vi "DataProcessingDraft.vi"() -> ()   [LabVIEW 2011]
uses:
  olin-sail-bot/Software/2-Think/2 Typedefs/logger data.ctl
  olin-sail-bot/Software/2-Think/2 Typedefs/Which Boat.ctl
  olin-sail-bot/Software/2-Think/2 Typedefs/UTM Location.ctl
  olin-sail-bot/Software/2-Think/2 Typedefs/heading.ctl
  olin-sail-bot/Software/2-Think/2 Typedefs/rate of turn.ctl
  olin-sail-bot/Software/2-Think/2 Typedefs/robot velocity.ctl
  olin-sail-bot/Software/2-Think/2 Typedefs/pitch and roll.ctl
  olin-sail-bot/Software/2-Think/2 Typedefs/generalized sensor status.ctl
  olin-sail-bot/Software/2-Think/2 Typedefs/indicator LED.ctl
  olin-sail-bot/Software/2-Think/2 Typedefs/apparent wind direction.ctl
  olin-sail-bot/Software/2-Think/2 Typedefs/apparent wind speed.ctl
  olin-sail-bot/Software/2-Think/2 Typedefs/absolute wind direction.ctl
  olin-sail-bot/Software/2-Think/2 Typedefs/absolute wind speed.ctl
  olin-sail-bot/Software/0x2-OCU-Think Comm/0x2 Typedefs/Current Waypoint.ctl
  olin-sail-bot/Software/2-Think/2 Typedefs/UTM Circle.ctl
  olin-sail-bot/Software/2-Think/2 Typedefs/rudder angle.ctl
  olin-sail-bot/Software/2-Think/2 Typedefs/sail setpt.ctl
  olin-sail-bot/Software/0x2-OCU-Think Comm/0x2 Typedefs/manual override.ctl
  olin-sail-bot/Software/2-Think/2 Typedefs/setpoints to boat.ctl
panel:
  in  "Stop Viewing Data":bool
  in  "Choose graph to display":T1(tab)
  in  "Max Frequency":dbl
  out "Code Speed":cluster{i32[], dbl[]}[](graph)
  out "Battery Voltage":cluster{i32[], dbl[]}(graph)
  in  "Max Velocity":dbl
  out "Velocity":cluster{i32[], dbl[]}[](graph)
  in  "Max Angle":dbl
  out "Headings":cluster{i32[], dbl[]}[](graph)
  out "Rudder":cluster{i32[], dbl[]}(graph)
  out "Sail":cluster{i32[], dbl[]}(graph)
  in  "Data Log":T2 {"Current Waypoint Coords"."North" format="%#_10f"; "Current Waypoint Coords"."East" format="%#_8f"; "Robot Pitch/Roll"."Roll" format="%05.1f"; "Robot Pitch/Roll"."Pitch" format="%05.1f"; "Robot\nRate of Turn" format="%05.1f"; "Robot\nHeading" format="%05.1f"; "Robot UTM Location"."North" format="%#_10f"; "Robot UTM Location"."East" format="%#_8f"}
  # "Act and network frequency are always 0.\nAs far as I can tell, network frequency is never set, so of course it's 0.\nAct, while set, is in a sequence structure where the first frame has a while loop that only ends if we e-stop, so it'll never get set."
  # "Where Am I?"
  # "Path Planning"
  # "From Planning Functions"
  # "(this is not a cluster because subitems\nare generated in parallel code)"
  # "How Am I?"
  # "What's Around Me?"
  # "As Measured"
  # "As Measured"
  # "Loop Rates"
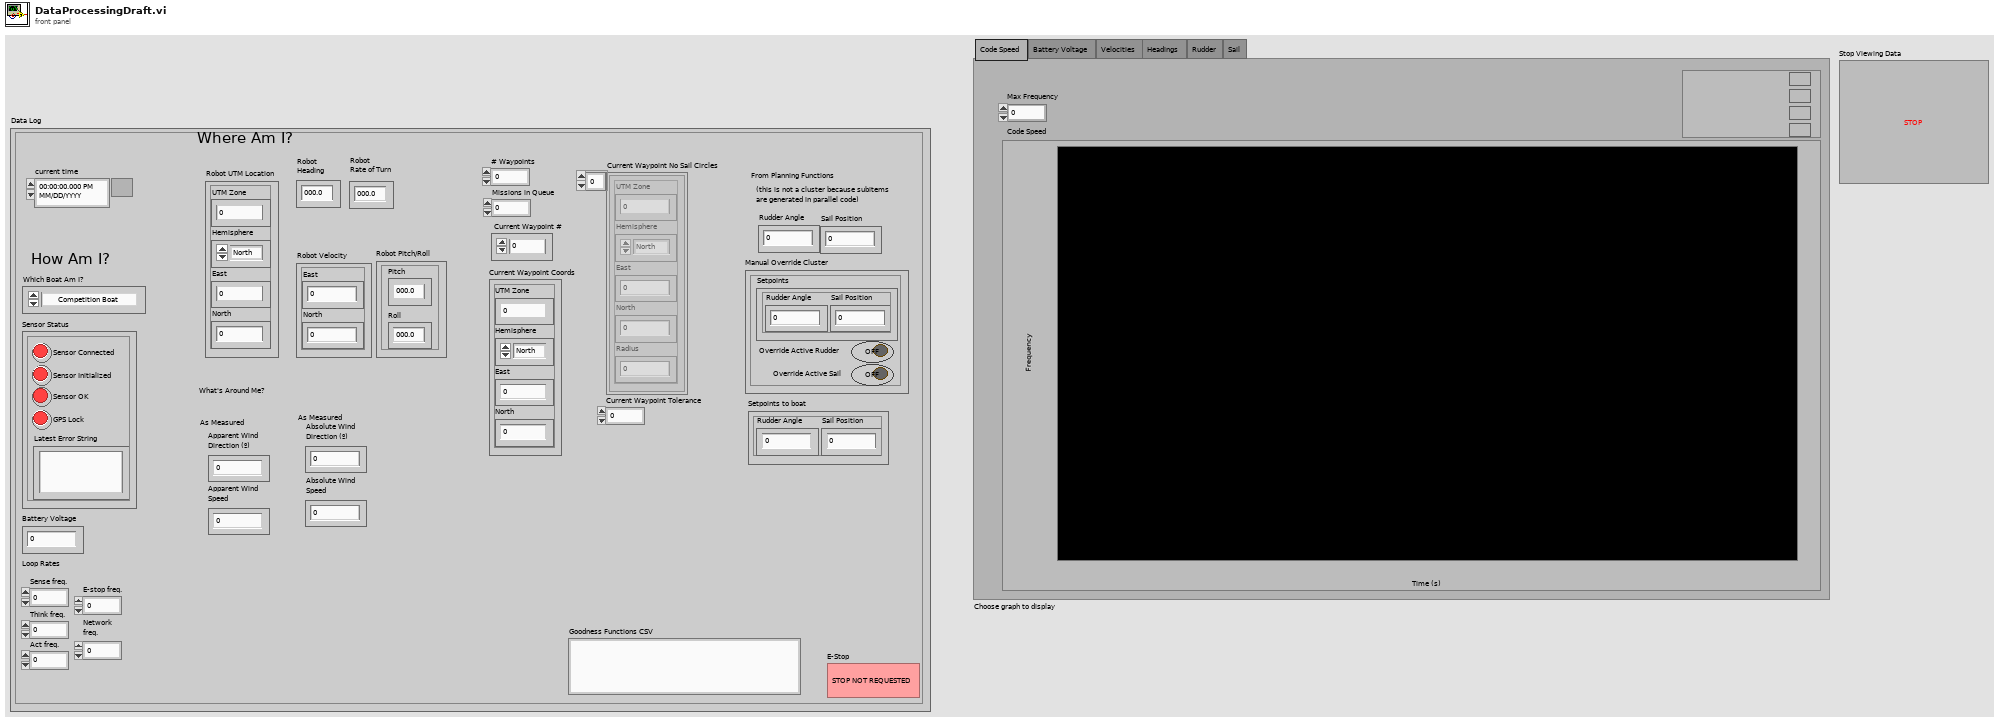
[diagram p1: front panel]
types:
  T1 = enum32{"Code Speed", "Battery Voltage", "Velocities", "Headings", "Rudder", "Sail"}
  T2 = typedef "logger data.ctl" = cluster{"current time":timestamp, "Which Boat Am I?":T3, "Robot UTM Location":T4, "Robot\nHeading ":T5, "Robot\nRate of Turn":T6, "Robot Velocity":T7, "Robot Pitch/Roll":T8, "Sensor Status":T9, "Battery Voltage":dbl, "Sense freq.":dbl, "Think freq.":dbl, "Act freq.":dbl, "E-stop freq.":dbl, "Network \nfreq.":dbl, "Apparent Wind\nDirection (º)":T11, "Apparent Wind\nSpeed":T12, "Absolute Wind\nDirection (º)":T13, "Absolute Wind\nSpeed":T14, "Missions in Queue":i32, "# Waypoints":i32, " Current Waypoint #":T15, "Current Waypoint Coords":T4, "Current Waypoint Tolerance":dbl, "Current Waypoint No Sail Circles":T16[], "Rudder Angle":T17, "Sail Position":T18, "Manual Override Cluster":T19, "Setpoints to boat":T20, "E-Stop":bool, "Goodness Functions CSV":string}
  T3 = typedef "Which Boat.ctl" = enum16{"Competition Boat", "Small RC", "Simulation"}
  T4 = typedef "UTM Location.ctl" = cluster{"UTM Zone":dbl, "Hemisphere":enum16{"North", "South"}, "East":dbl, "North":dbl}
  T5 = typedef "heading.ctl" = dbl
  T6 = typedef "rate of turn.ctl" = dbl
  T7 = typedef "robot velocity.ctl" = cluster{"East":dbl, "North":dbl}
  T8 = typedef "pitch and roll.ctl" = cluster{"Pitch":dbl, "Roll":dbl}
  T9 = typedef "generalized sensor status.ctl" = cluster{"Sensor Connected":T10, "Sensor Initialized":T10, "Sensor OK":T10, "Latest Error String":string, "GPS Lock":T10}
  T10 = typedef "indicator LED.ctl" = bool
  T11 = typedef "apparent wind direction.ctl" = dbl
  T12 = typedef "apparent wind speed.ctl" = dbl
  T13 = typedef "absolute wind direction.ctl" = dbl
  T14 = typedef "absolute wind speed.ctl" = dbl
  T15 = typedef "Current Waypoint.ctl" = i32
  T16 = typedef "UTM Circle.ctl" = cluster{"UTM Zone":dbl, "Hemisphere":enum16{"North", "South"}, "East":dbl, "North":dbl, "Radius":dbl}
  T17 = typedef "rudder angle.ctl" = dbl
  T18 = typedef "sail setpt.ctl" = dbl
  T19 = typedef "manual override.ctl" = cluster{"Override Active Rudder":bool, "Setpoints":T20, "Override Active Sail":bool}
  T20 = typedef "setpoints to boat.ctl" = cluster{"Sail Position":T18, "Rudder Angle":T17}
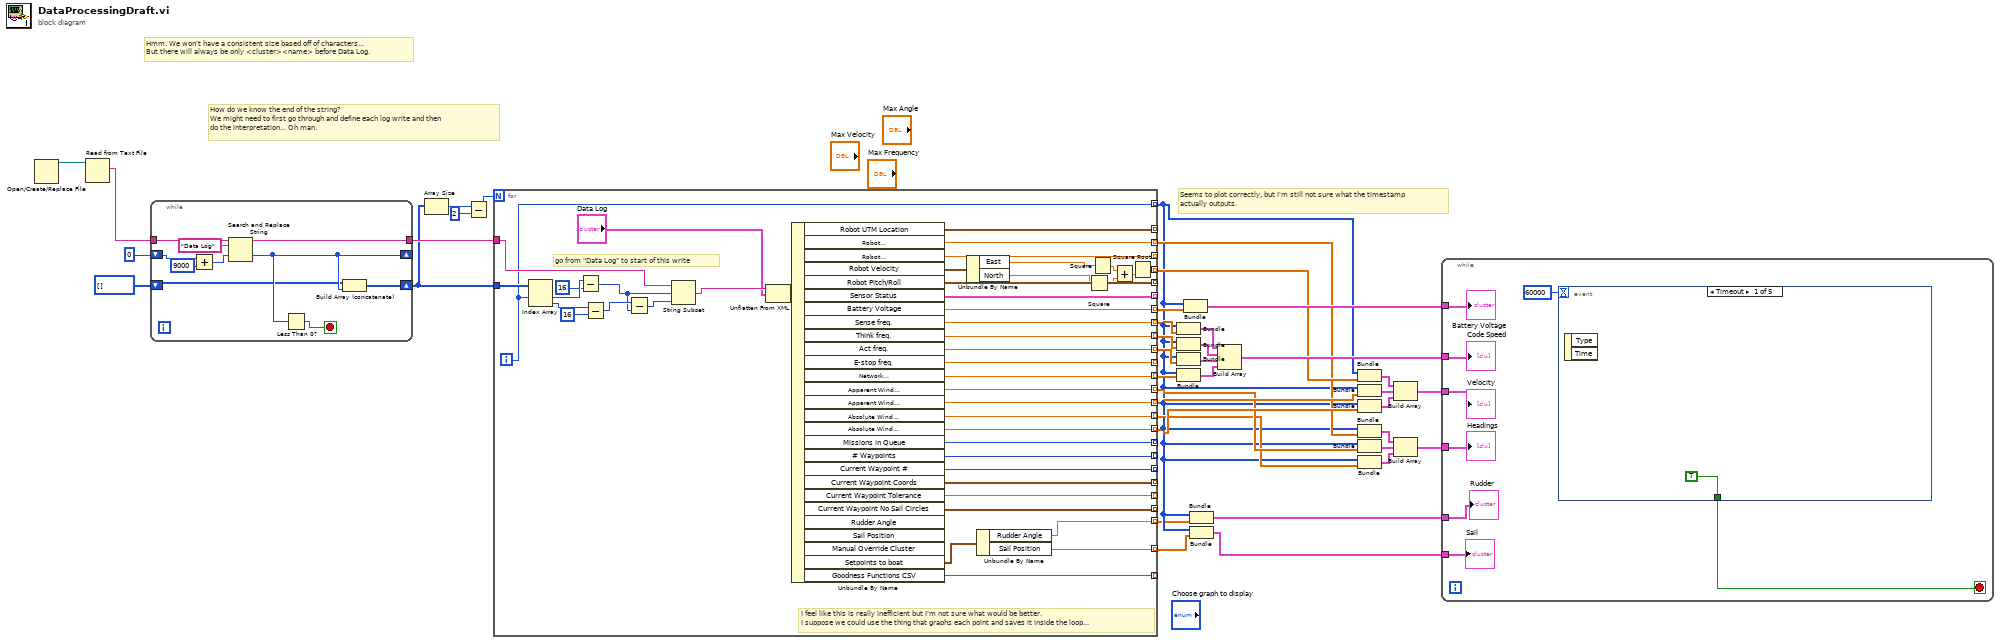
[diagram p0: block diagram]
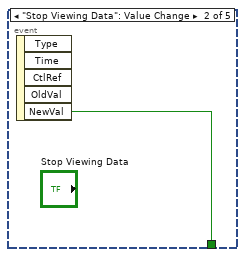
[diagram p2: hidden frame]
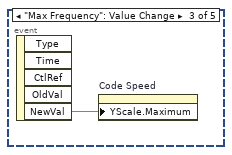
[diagram p3: hidden frame]
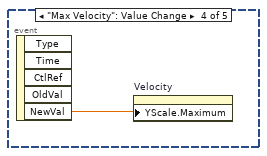
[diagram p4: hidden frame]
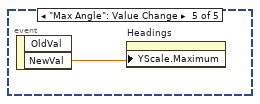
[diagram p5: hidden frame]
diagram:
  # "Seems to plot correctly, but I'm still not sure what the timestamp\nactually outputs."
  # "How do we know the end of the string?\nWe might need to first go through and define each log write and then\ndo the interpretation... Oh man."
  # "Hmm. We won't have a consistent size based off of characters...\nBut there will always be only <cluster><name> before Data Log."
  n1 = Open/Create/Replace File() -> (refnum out=w39:refnum<file>)  [unwired: 6 in, 2 out]
  n2 = Read from Text File(file (use dialog)=w39) -> (text=w38:string)  [unwired: 3 in, 3 out]
  n3 = while {
    tunnel: w38 -> [w48]
    shift-right: [w43] -> _
    shift-left: 0 ("offset past replacement") -> [w47]
    shift-right: [w42] -> w34
    shift-left: i32[] [] -> [w41]
    tunnel: [w40] -> w35
    stop <- w44 stop-if-true
    n4 = Add(x=w47, y=9000) -> (x+y=w45:i32)
    n5 = Search and Replace String(input string=w48, search string="Data Log", offset=w45) -> (result string=w40:string, offset past replacement=w43:i32)  [unwired: 5 in, 2 out]
    n6 = Less Than 0?(x=w43) -> (x < 0?=w44:bool)
    n7 = Build Array (concatenate)(w41, w43) -> (w42:i32[])
  }
  n8 = Array Size(array=w34) -> (size(s)=w33:i32)
  n9 = Subtract(x=w33, y=2) -> (x-y=w32:i32)
  n10 = for {
    N: w32 -> [_]
    tunnel: w34 -> [w86]
    tunnel: w35 -> [w89]
    tunnel: [w82] -> _ mode=indexing
    tunnel: [w81] -> w9 mode=indexing
    tunnel: [w80] -> _ mode=indexing
    tunnel: [w79] -> _ mode=indexing
    tunnel: [w78] -> _ mode=indexing
    tunnel: [w77] -> w20 mode=indexing
    tunnel: [w76] -> w18 mode=indexing
    tunnel: [w75] -> w17 mode=indexing
    tunnel: [w74] -> w16 mode=indexing
    tunnel: [w73] -> _ mode=indexing
    tunnel: [w72] -> w15 mode=indexing
    tunnel: [w71] -> w8 mode=indexing
    tunnel: [w70] -> w12 mode=indexing
    tunnel: [w69] -> w7 mode=indexing
    tunnel: [w68] -> w11 mode=indexing
    tunnel: [w67] -> _ mode=indexing
    tunnel: [w66] -> _ mode=indexing
    tunnel: [w65] -> _ mode=indexing
    tunnel: [w64] -> _ mode=indexing
    tunnel: [w63] -> _ mode=indexing
    tunnel: [w62] -> _ mode=indexing
    tunnel: [w61] -> _ mode=indexing
    tunnel: [w60] -> w6 mode=indexing
    tunnel: [w53] -> w13 mode=indexing
    tunnel: [w51] -> w4 mode=indexing
    tunnel: [w50] -> w3 mode=indexing
    i -> [w60]
    # "I feel like this is really inefficient but I'm not sure what would be better.\nI suppose we could use the thing that graphs each point and saves it inside the loop..."
    # "go from \"Data Log\" to start of this write"
    n11 = Index Array(array=w86, index #1=w60) -> (element #1=w94:i32, element #2=w92:i32)  [unwired: 1 in]
    n12 = Subtract(x=w94, y=16) -> (x-y=w87:i32)
    n13 = Subtract(x=w92, y=16) -> (x-y=w90:i32)
    n14 = Subtract(x=w90, y=w87) -> (x-y=w88:i32)
    n15 = String Subset(string=w89, offset (0)=w87, length (rest)=w88) -> (substring=w85:string)
    n16 = Unflatten From XML(xml string=w85, type="Data Log") -> (value=w83:T2)  [unwired: 1 in, 1 out]
    n17 = Unbundle By Name(w83) -> ("Robot UTM Location"=w82:T4, "Robot\nHeading"=w81:T5, "Robot\nRate of Turn"=w80:T6, "Robot Velocity"=w59:T7, "Robot Pitch/Roll"=w79:T8, "Sensor Status"=w78:T9, "Battery Voltage"=w77:dbl, "Sense freq."=w76:dbl, "Think freq."=w75:dbl, "Act freq."=w74:dbl, "E-stop freq."=w73:dbl, "Network \nfreq."=w72:dbl, "Apparent Wind\nDirection (º)"=w71:T11, "Apparent Wind\nSpeed"=w70:T12, "Absolute Wind\nDirection (º)"=w69:T13, "Absolute Wind\nSpeed"=w68:T14, "Missions in Queue"=w67:i32, "# Waypoints"=w66:i32, "Current Waypoint #"=w65:T15, "Current Waypoint Coords"=w64:T4, "Current Waypoint Tolerance"=w63:dbl, "Current Waypoint No Sail Circles"=w62:T16[], "Setpoints to boat"=w52:T20, "Goodness Functions CSV"=w61:string)  [unwired: 3 out]
    n18 = Unbundle By Name(w59) -> ("East"=w58:dbl, "North"=w57:dbl)
    n19 = Unbundle By Name(w52) -> ("Rudder Angle"=w51:T17, "Sail Position"=w50:T18)
    n20 = Square(x=w57) -> (x^2=w54:dbl)
    n21 = Square(x=w58) -> (x^2=w55:dbl)
    n22 = Add(x=w55, y=w54) -> (x+y=w56:dbl)
    n23 = Square Root(x=w56) -> (sqrt(x)=w53:dbl)
  }
  n24 = Bundle(w6, w18) -> (w22:cluster{i32[], dbl[]})  [unwired: 1 in]
  n25 = Bundle(w6, w17) -> (w21:cluster{i32[], dbl[]})  [unwired: 1 in]
  n26 = Bundle(w6, w16) -> (w24:cluster{i32[], dbl[]})  [unwired: 1 in]
  n27 = Bundle(w6, w15) -> (w23:cluster{i32[], dbl[]})  [unwired: 1 in]
  n28 = Bundle(w6, w20) -> (w19:cluster{i32[], dbl[]})  [unwired: 1 in]
  n29 = Bundle(w6, w4) -> (w2:cluster{i32[], T17[]})  [unwired: 1 in]
  n30 = Bundle(w6, w3) -> (w1:cluster{i32[], T18[]})  [unwired: 1 in]
  n31 = Build Array(w22, w21, w24, w23) -> (w14:cluster{i32[], dbl[]}[])
  n32 = Bundle(w6, w13) -> (w28:cluster{i32[], dbl[]})  [unwired: 1 in]
  n33 = Bundle(w6, w12) -> (w29:cluster{i32[], T12[]})  [unwired: 1 in]
  n34 = Bundle(w6, w11) -> (w30:cluster{i32[], T14[]})  [unwired: 1 in]
  n35 = Bundle(w6, w9) -> (w25:cluster{i32[], T5[]})  [unwired: 1 in]
  n36 = Bundle(w6, w8) -> (w26:cluster{i32[], T11[]})  [unwired: 1 in]
  n37 = Bundle(w6, w7) -> (w27:cluster{i32[], T13[]})  [unwired: 1 in]
  n38 = Build Array(w28, w29, w30) -> (w10:cluster{i32[], T14[]}[])
  n39 = Build Array(w25, w26, w27) -> (w5:cluster{i32[], T13[]}[])
  n40 = while {
    tunnel: w19 -> [w102]
    tunnel: w14 -> [w101]
    tunnel: w10 -> [w100]
    tunnel: w5 -> [w99]
    tunnel: w2 -> [w96]
    tunnel: w1 -> [w95]
    stop <- w97 stop-if-true
    n41 = event shown="[0] Timeout" {
      selector: _ -> [_ _ _ _ _]
      dyn-events: _ -> [_ _ _ _ _]
      timeout: 60000 -> [_ _ _ _ _]
      tunnel: [TRUE w104 _ _ _] -> w97
      event Timeout {
        n42 = event-data() -> ()  [unwired: 1 in, 2 out]
      }
      event "Stop Viewing Data": Value Change {
        n43 = event-data() -> ("NewVal"=w104:bool)  [unwired: 1 in, 4 out]
      }
      event "Max Frequency": Value Change {
        n44 = event-data() -> ("NewVal"=w105:dbl)  [unwired: 1 in, 4 out]
        n45 = property on="Code Speed" class="XYGraph (strict)"("YScale.Maximum"=w105) -> ()  [unwired: 2 in, 2 out]
      }
      event "Max Velocity": Value Change {
        n46 = event-data() -> ("NewVal"=w106:dbl)  [unwired: 1 in, 4 out]
        n47 = property on="Velocity" class="XYGraph (strict)"("YScale.Maximum"=w106) -> ()  [unwired: 2 in, 2 out]
      }
      event "Max Angle": Value Change {
        n48 = event-data() -> ("NewVal"=w107:dbl)  [unwired: 1 in, 1 out]
        n49 = property on="Headings" class="XYGraph (strict)"("YScale.Maximum"=w107) -> ()  [unwired: 2 in, 2 out]
      }
    }
    "Velocity" <- w100
    "Rudder" <- w96
    "Headings" <- w99
    "Code Speed" <- w101
    "Battery Voltage" <- w102
    "Sail" <- w95
  }
